vi "Add Resource (Tx DSP).vi"(0 "niUSRP Tx DSP v2 FPGA.lvclass":refnum<class "niUSRP Tx DSP v2 FPGA.lvclass">, 1 "instance (0)":u8) -> (4 "niUSRP Tx DSP v2 FPGA.lvclass 2":refnum<class "niUSRP Tx DSP v2 FPGA.lvclass">)   [LabVIEW 2025, in "niUSRP Tx DSP v2 FPGA.lvclass"]
uses:
  niUSRP Tx DSP v2 FPGA.lvclass
  niUSRP Tx DSP v2 FPGA.lvclass/niUSRP Tx DSP v2 FPGA.ctl
  <vilib>/rvi/DataTransferAndStorage/Container/Common/niFpgaContainerGetUniqueNameForEmu.vi
  <vilib>/rvi/DataTransferAndStorage/Container/Common/niFpgaContainerSetEmuInfo.vi
  <vilib>/rvi/eio/common/nirviEmuReportErrorAndStop.vi
  <vilib>/rvi/LocalResourceManager/LocalResourceManager.xnode
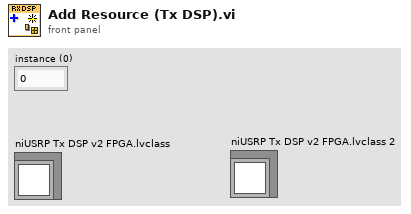
[diagram p1: front panel]
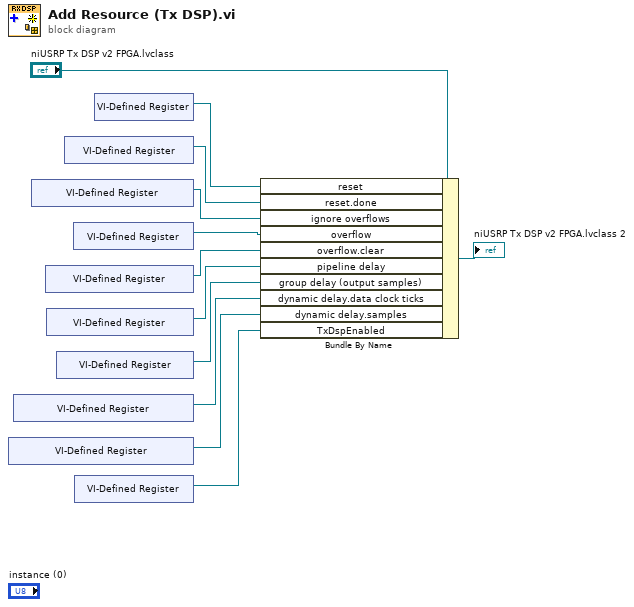
[diagram p0: block diagram]
diagram:
  n1 = xnode "VI-Defined Register"() -> ("Register Out"=w3:refnum<k21>)
  n2 = xnode "VI-Defined Register"() -> ("Register Out"=w2:refnum<k21>)
  n3 = xnode "VI-Defined Register"() -> ("Register Out"=w6:refnum<k21>)
  n4 = xnode "VI-Defined Register"() -> ("Register Out"=w8:refnum<k21>)
  n5 = xnode "VI-Defined Register"() -> ("Register Out"=w5:refnum<k21>)
  n6 = xnode "VI-Defined Register"() -> ("Register Out"=w4:refnum<k21>)
  n7 = xnode "VI-Defined Register"() -> ("Register Out"=w9:refnum<k21>)
  n8 = xnode "VI-Defined Register"() -> ("Register Out"=w7:refnum<k21>)
  n9 = xnode "VI-Defined Register"() -> ("Register Out"=w1:refnum<k21>)
  n10 = xnode "VI-Defined Register"() -> ("Register Out"=w10:refnum<k21>)
  n11 = Bundle By Name(cluster="niUSRP Tx DSP v2 FPGA.lvclass", "reset"=w10, "reset.done"=w9, "ignore overflows"=w6, "overflow"=w7, "overflow.clear"=w8, "pipeline delay"=w5, "group delay (output samples)"=w4, "dynamic delay.data clock ticks"=w2, "dynamic delay.samples"=w3, "TxDspEnabled"=w1) -> (→"niUSRP Tx DSP v2 FPGA.lvclass 2":refnum<class "niUSRP Tx DSP v2 FPGA.lvclass">)
